vi "c_Wait for Client.vi"() -> (1 "Case Label":T1="Wait for Client")   [LabVIEW 2020, in "Listener.lvclass"]
uses:
  <vilib>/addons/_Workers/Library/Case Label.ctl
  Listener.lvclass
  <vilib>/addons/_Workers/Library/Workers.lvlib
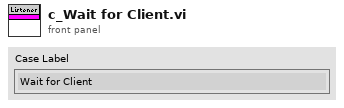
[diagram p1: front panel]
types:
  T1 = typedef "Workers.lvlib/Case Label.ctl" = string
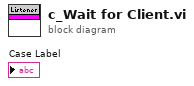
[diagram p0: block diagram]
diagram:
